vi "Afstand.vi"() -> ()   [LabVIEW 2018]
panel:
  out "analog in":dbl[](array[numeric]) format="%0.2f"
  in  "stop":bool
  out "Afstand":bool
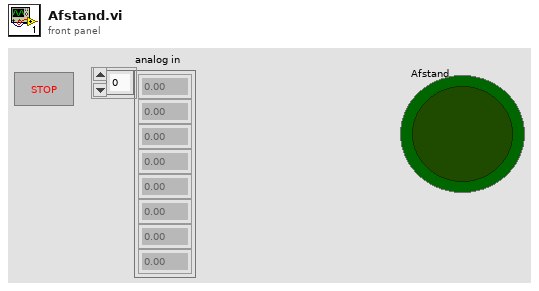
[diagram p1: front panel]
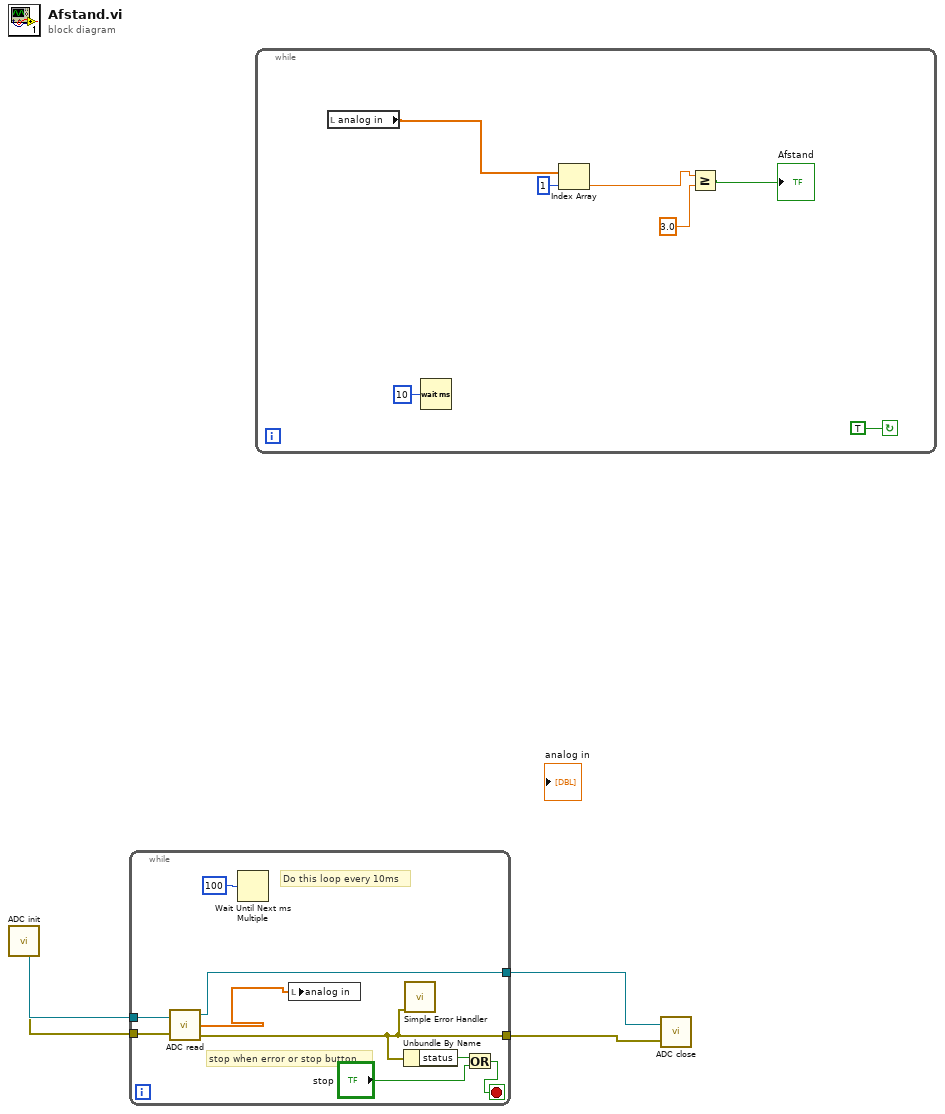
[diagram p0: block diagram]
diagram:
  n1 = call "ADC init.vi"() -> ("error out"=w3:errorcluster, "task out"=w4:refnum<k21>)
  n2 = while {
    tunnel: w4 -> [w13]
    tunnel: w3 -> [w12]
    tunnel: [w9] -> w2
    tunnel: [w11] -> w1
    stop <- w6 stop-if-true
    # "stop when error or stop button"
    # "Do this loop every 10ms"
    n3 = call "ADC read.vi"("task/channels in"=w13, "error in"=w12) -> ("task out"=w11:refnum<k21>, "analog in"=w5:dbl[], "error out"=w9:errorcluster)
    n4 = Wait Until Next ms Multiple(millisecond multiple=u32 100) -> ()  [unwired: 1 out]
    n5 = local write "analog in"(w5) -> ()
    n6 = Unbundle By Name(w9) -> ("status"=w8:bool)
    n7 = call <vilib>:"Simple Error Handler.vi"("error in (no error)"=w9) -> ()  [unwired: 4 in, 5 out]
    n8 = Or(x=w8, y="stop") -> (x .or. y?=w6:bool)
  }
  n9 = while {
    stop <- TRUE continue-if-true
    n10 = local read "analog in"() -> (w14:dbl[])
    n11 = Wait (ms)(milliseconds to wait=u32 10) -> ()  [unwired: 1 out]
    n12 = Index Array(array=w14, index=1) -> (element=w18:dbl)
    n13 = Greater Or Equal?(x=w18, y=3.0) -> (x >= y?=→"Afstand":bool)
  }
  n14 = call "ADC close.vi"("error in"=w2, "task/channels in"=w1) -> ()
